vi "PressureReadout.vi"(0 "error in":errorcluster, 4 "PT3 Pin":u16, 6 "PT2 Pin":u16, 8 "Handle In":i32, 9 "PT1 Pin":u16) -> (1 "PT3 Voltage Reading":dbl, 2 "PT3 Pressure Reading":dbl, 3 "error out":errorcluster[](array[cluster]), 5 "PT2 Pressure Reading":dbl, 7 "PT2 Voltage Reading":dbl, 10 "PT1 Voltage Reading":dbl, 11 "PT1 Pressure Reading":dbl)   [LabVIEW 2021]
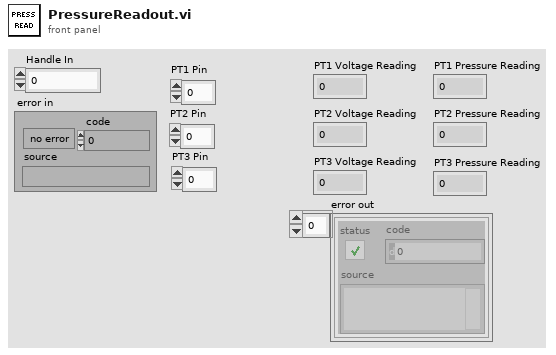
[diagram p1: front panel]
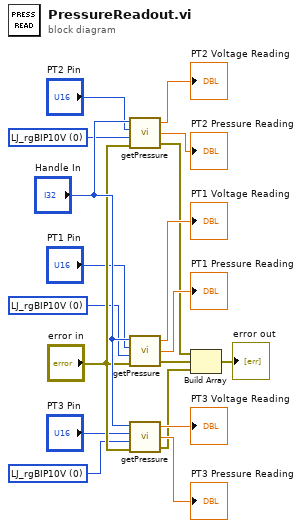
[diagram p0: block diagram]
diagram:
  w14 = u16 0 items=["LJ_rgBIP10V", "LJ_rgBIP1V", "LJ_rgBIPP1V", "LJ_rgBIPP01V"] ("AIN Range")
  w15 = u16 0 items=["LJ_rgBIP10V", "LJ_rgBIP1V", "LJ_rgBIPP1V", "LJ_rgBIPP01V"] ("AIN Range")
  w16 = u16 0 items=["LJ_rgBIP10V", "LJ_rgBIP1V", "LJ_rgBIPP1V", "LJ_rgBIPP01V"] ("AIN Range")
  n1 = call "getPressure.vi"("error in"="error in", "AIN Range"=w15, "+Channel"="PT2 Pin", "Handle In"="Handle In") -> ("error out"=w2:errorcluster, "Pressure Reading"=→"PT2 Pressure Reading":dbl, "Voltage Reading"=→"PT2 Voltage Reading":dbl)
  n2 = call "getPressure.vi"("error in"="error in", "AIN Range"=w14, "+Channel"="PT1 Pin", "Handle In"="Handle In") -> ("error out"=w3:errorcluster, "Pressure Reading"=→"PT1 Pressure Reading":dbl, "Voltage Reading"=→"PT1 Voltage Reading":dbl)
  n3 = call "getPressure.vi"("error in"="error in", "AIN Range"=w16, "+Channel"="PT3 Pin", "Handle In"="Handle In") -> ("error out"=w4:errorcluster, "Pressure Reading"=→"PT3 Pressure Reading":dbl, "Voltage Reading"=→"PT3 Voltage Reading":dbl)
  n4 = Build Array(w2, w3, w4) -> (→"error out":errorcluster[])
